vi "boundingBoxCoords.vi"(10 "side length (px)":i32, 11 "center (x,y)":i32[](array[numeric])) -> (2 "bounding rectangle":i32[](array[numeric]), 3 "bounding box":T1)   [LabVIEW 2015]
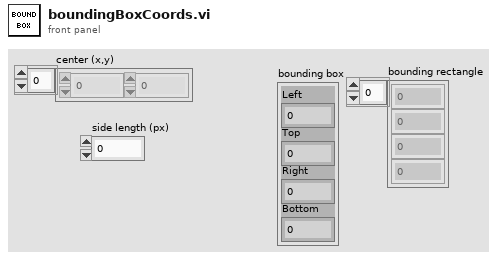
[diagram p1: front panel]
types:
  T1 = cluster{"Left":i32, "Top":i32, "Right":i32, "Bottom":i32}
  T2 = cluster{"[0]":i32, "[1]":i32, "[2]":i32, "[3]":i32}
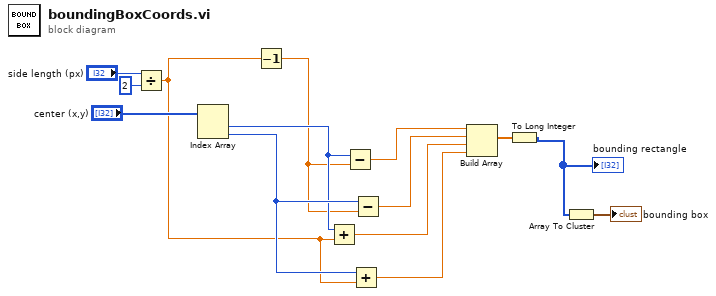
[diagram p0: block diagram]
diagram:
  n1 = Divide(x="side length (px)", y=2) -> (x/y=w1:dbl)
  n2 = Index Array(array="center (x,y)") -> (element #1=w10:i32, element #2=w11:i32)  [unwired: 2 in]
  n3 = Decrement(x=w1) -> (x-1=w2:dbl)
  n4 = Add(x=w10, y=w1) -> (x+y=w7:dbl)
  n5 = Subtract(x=w10, y=w2) -> (x-y=w9:dbl)
  n6 = Add(x=w11, y=w1) -> (x+y=w6:dbl)
  n7 = Subtract(x=w11, y=w2) -> (x-y=w8:dbl)
  n8 = Build Array(w9, w8, w7, w6) -> (w5:dbl[])
  n9 = To Long Integer(number=w5) -> (32bit integer=w4:i32[])
  "bounding rectangle" <- w4
  n10 = Array To Cluster(array=w4) -> (cluster=→"bounding box":T2)
